vi "run top level.vi"(11 "task":refnum<class "task.lvclass">) -> ()   [LabVIEW 2013, in "task.lvclass"]
uses:
  task/task.lvclass
  task/task.lvclass/task.ctl
  results reporter/results reporter.lvclass
  result/result.lvclass
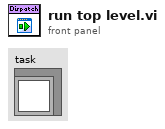
[diagram p1: front panel]
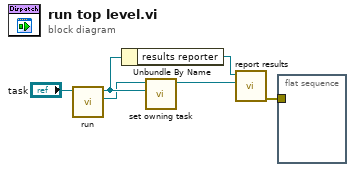
[diagram p0: block diagram]
diagram:
  n1 = call-dynamic "run.vi"("task in"="task") -> ("result"=w2:refnum<class "result.lvclass">, "task out"=w3:refnum<class "task.lvclass">)  [unwired: 9 in]
  n2 = Unbundle By Name(w3) -> ("results reporter"=w5:refnum<class "results reporter.lvclass">)
  n3 = call "set owning task.vi"("task"=w3, "result in"=w2) -> ("result out"=w1:refnum<class "result.lvclass">)  [unwired: 9 in]
  n4 = call-dynamic "report results.vi"("result"=w1, "results reporter in"=w5) -> ("error out"=w4:errorcluster)  [unwired: 8 in, 1 out]
  n5 = flat-sequence {
    tunnel: w4 -> [_]
    frame #0 {
    }
  }
